vi "Configure Reporting.vi"(8 "error in (no error)":errorcluster, 9 "Autogenerate?":bool=TRUE, 10 "Path":path, 11 "Execution API In":refnum<class "Execution API.lvclass">) -> (0 "error out":errorcluster, 3 "Execution API Out":refnum<class "Execution API.lvclass">)   [LabVIEW 2020, in "Execution API.lvclass"]
doc: "Configure reporting path and turn on automatic report generation."
uses:
  Execution API.lvclass
  Execution API.lvclass/Execution API.ctl
  Report Generator/Report Generator.lvclass
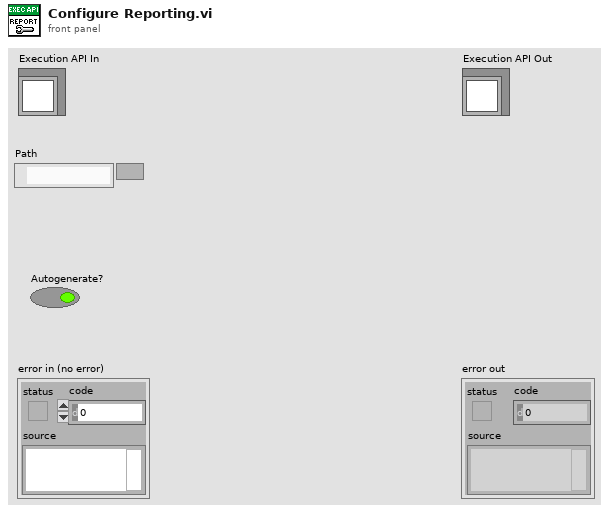
[diagram p1: front panel]
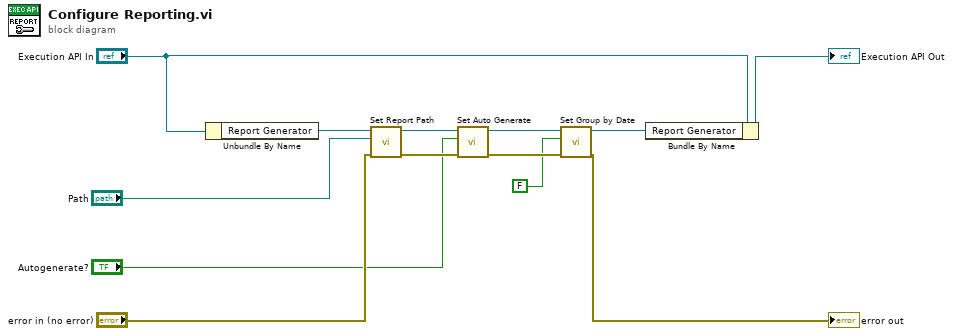
[diagram p0: block diagram]
diagram:
  n1 = Unbundle By Name("Execution API In") -> ("Report Generator"=w8:refnum<class "Report Generator.lvclass">)
  n2 = call "Set Report Path.vi"("error in (no error)"="error in (no error)", "Path"="Path", "Report Generator In"=w8) -> ("error out"=w11:errorcluster, "Report Generator Out"=w9:refnum<class "Report Generator.lvclass">)  [unwired: 7 in]
  n3 = call "Set Auto Generate.vi"("error in (no error)"=w11, "Autogenerate?"="Autogenerate?", "Report Generator In"=w9) -> ("error out"=w3:errorcluster, "Report Generator Out"=w5:refnum<class "Report Generator.lvclass">)  [unwired: 7 in]
  n4 = call "Set Group by Date.vi"("error in (no error)"=w3, "Group by Date?"=FALSE, "Report Generator In"=w5) -> ("error out"=→"error out":errorcluster, "Report Generator Out"=w4:refnum<class "Report Generator.lvclass">)  [unwired: 7 in]
  n5 = Bundle By Name(cluster="Execution API In", "Report Generator"=w4) -> (→"Execution API Out":refnum<class "Execution API.lvclass">)
